vi "Keyence_写入多个寄存器数据.vi"(0 "Keyence ID In":refnum<k5>, 1 "Delay Time (s)":dbl=1.0 caption="延迟时间(s)", 5 "软元件编号":string, 9 "值组":string[](array[string]), 11 "错误输入（无错误）":errorcluster) -> (4 "Keyence ID Out":refnum<k5>, 6 "数据输出":string, 8 "写入个数":string, 10 "状态":bool, 15 "错误输出":errorcluster)   [LabVIEW 2017]
panel:
  out "连接的字符串":string
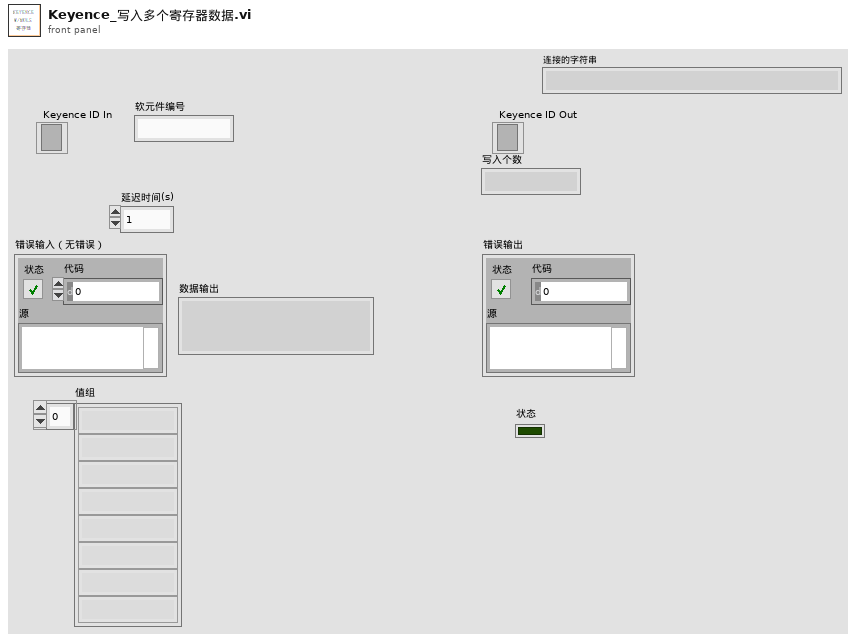
[diagram p1: front panel]
types:
  T1 = enum16{"Standard", "Buffered", "CRLF", "Immediate"}
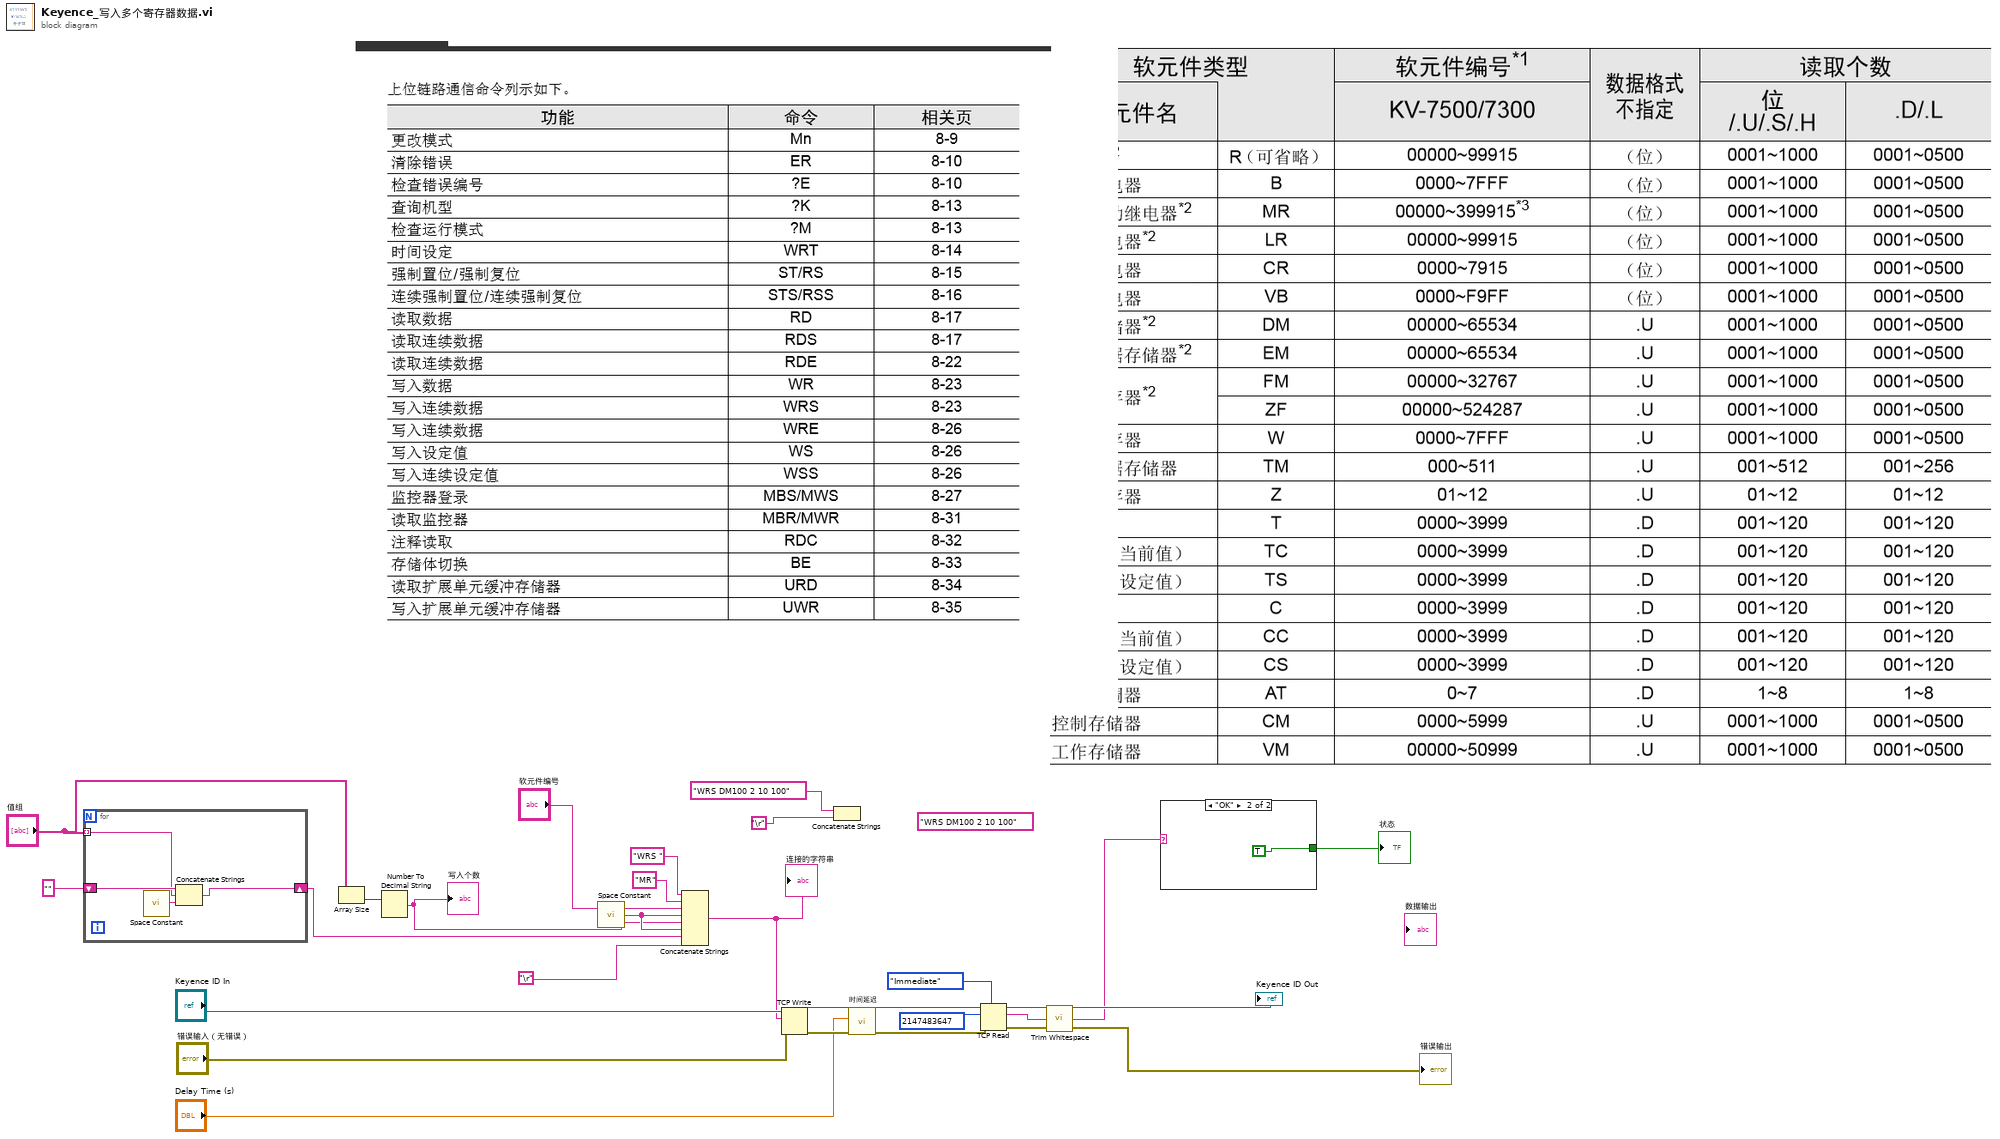
[diagram p0: block diagram]
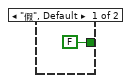
[diagram p2: hidden frame]
diagram:
  (unwired) "WRS DM100 2 10 100"
  n1 = for {
    tunnel: "值组" -> [w29] mode=indexing
    shift-right: [w27] -> w5
    shift-left: "" -> [w30]
    n2 = call <vilib>:"Space Constant.vi"() -> ("String"=w28:string)
    n3 = Concatenate Strings(w30, w29, w28) -> (w27:string)
  }
  n4 = Array Size(array="值组") -> (size(s)=w2:i32)
  n5 = Number To Decimal String(number=w2) -> (decimal integer string=w1:string)  [unwired: 1 in]
  "写入个数" <- w1
  n6 = call <vilib>:"Space Constant.vi"() -> ("String"=w3:string)
  n7 = Concatenate Strings("WRS ", "MR" ("字符串"), "软元件编号", w3, w1, w3, w5, "\r") -> (w12:string)
  "连接的字符串" <- w12
  n8 = TCP Write(connection ID="Keyence ID In", data in=w12, error in (no error)="错误输入（无错误）") -> (connection ID out=w24:refnum<k5>, error out=w23:errorcluster)  [unwired: 1 in, 1 out]
  n9 = Concatenate Strings("WRS DM100 2 10 100", "\r") -> ()  [unwired: 1 out]
  n10 = call "时间延迟"("error in (no error)"=w23, "Delay Time (s)"="Delay Time (s)") -> ("error out"=w18:errorcluster)  [unwired: 9 in]
  n11 = TCP Read(connection ID=w24, bytes to read=2147483647 ("读取的字节"), error in (no error)=w18, 7:T1."Immediate" ("模式（标准）")) -> (connection ID out=→"Keyence ID Out":refnum<k5>, data out=w9:string, error out=→"错误输出":errorcluster)  [unwired: 1 in]
  n12 = call <vilib>:"Trim Whitespace.vi"("string"=w9) -> ("trimmed string"=w8:string)  [unwired: 1 in]
  n13 = case shown="\"OK\"" w8 {
    tunnel: [FALSE TRUE] -> w7
    frame "假", Default {
    }
    frame "OK" {
    }
  }
  "状态" <- w7
